vi "Gen mnu.vi"(8 "error in (no error)":errorcluster, 11 "Progress":refnum<vi>) -> (0 "error out":errorcluster, 3 "Progress (out)":refnum<vi>)   [LabVIEW 2020, in "WebServiceImporter.lvlib" / "VI Generator.lvlib"]
uses:
  <vilib>/Platform/WebService/VI Generator/VI Generator.lvlib
  <vilib>/Palette API/Palette Menu/Public Type Define/Palette type.ctl
  <vilib>/Palette API/Palette Menu/Public Type Define/Item.ctl
  <vilib>/Platform/WebService/Global/Const Strings.vi
  <resource>/importtools/Common/Icon/NISAST VI.Icon.lvclass
  <vilib>/Palette API/Palette Menu/Palette Menu.lvlib
  <vilib>/Platform/WebService/WebServiceImporter.lvlib
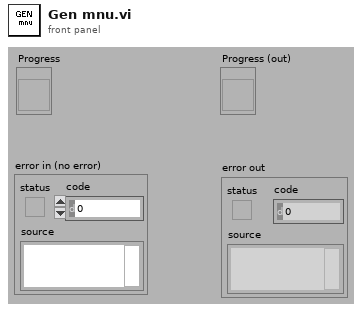
[diagram p1: front panel]
types:
  T1 = typedef "Palette Menu.lvlib/Item.ctl" = cluster{"item path":path, "library path":path, "use default lvlib palette":bool, "short name":string, "place VI contents":bool, "hide synchronized item":bool, "reserve spot for synch item":bool, "configure when placing VI contents":bool}
  T2 = typedef "Palette Menu.lvlib/Palette type.ctl" = i32
  T3 = typedef "Palette Menu.lvlib/Palette Data.ctl" = cluster{"display name":string, "view format":T4, "palette width":i16, "items":T5, "256 color icon":picture, "B&W color icon":picture, "help information":T6, "palette description":string, "synchronize information":T7}
  T4 = typedef "Palette Menu.lvlib/View Format.ctl" = u16
  T5 = typedef "Palette Menu.lvlib/Items.ctl" = T1[]
  T6 = typedef "Palette Menu.lvlib/Help Info.ctl" = cluster{"help tag":string, "help file path ":path}
  T7 = typedef "Palette Menu.lvlib/Synchronize Info.ctl" = cluster{"synchronize with directory":bool, "synchronize directory path":path}
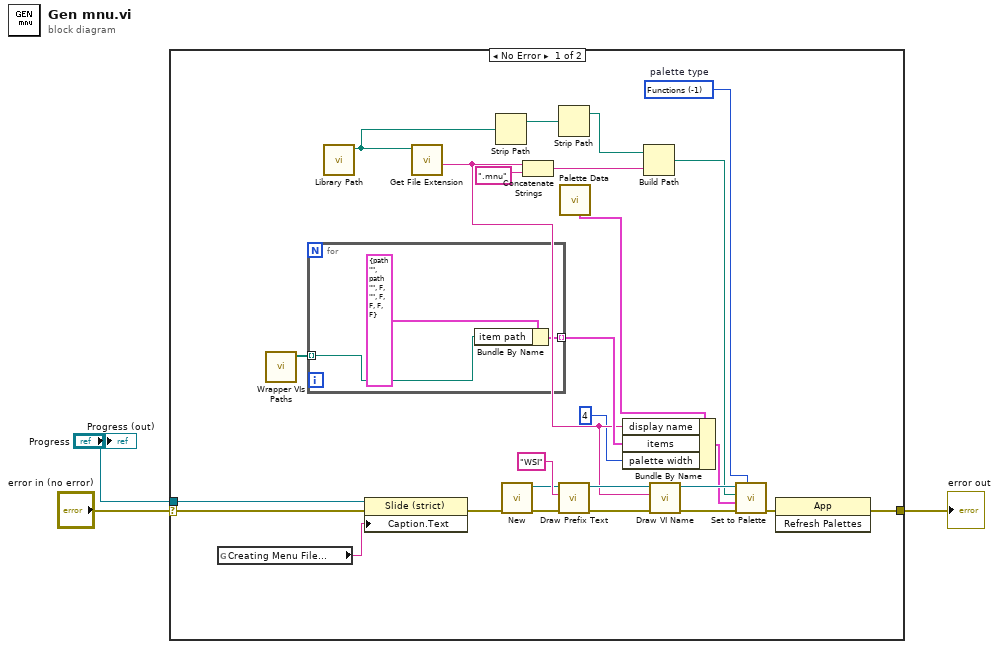
[diagram p0: block diagram]
diagram:
  n1 = case shown="No Error" "error in (no error)" {
    selector: "error in (no error)" -> [w4 w33]
    tunnel: [w14 w33] -> w3
    tunnel: "Progress" -> [w6 _]
    frame No Error {
      w16 = T2 -1 items=["Functions"=-1, "Controls"=-2]  # palette type
      n2 = global read "Const Strings.vi" "Creating Menu File..."() -> (w7:string)
      n3 = call <vilib>:"Wrapper VIs Paths.vi"() -> ("Array"=w9:path[])  [unwired: 3 in, 8 out]
      n4 = for {
        tunnel: [w32] -> w29 mode=indexing
        tunnel: w9 -> [w30] mode=indexing
        n5 = Bundle By Name(cluster=T1 {"item path"=path "", "library path"=path "", "use default lvlib palette"=FALSE, "short name"="", "place VI contents"=FALSE, "hide synchronized item"=FALSE, "reserve spot for synch item"=FALSE, "configure when placing VI contents"=FALSE} ("Items"), "item path"=w30) -> (w32:T1)
      }
      n6 = call <vilib>:"Library Path.vi"() -> ("Path (out)"=w13:path)  [unwired: 3 in, 8 out]
      n7 = property class="Slide (strict)"(reference=w6, error in=w4, "Caption.Text"=w7) -> (error out=w5:errorcluster)  [unwired: 1 out]
      n8 = call <vilib>:"Get File Extension.vi"("file"=w13) -> ("filename without extension"=w12:string)  [unwired: 1 in, 9 out]
      n9 = Strip Path(path=w13) -> (stripped path=w11:path)  [unwired: 1 out]
      n10 = call <resource>:"New.vi"("error in (no error)"=w5) -> ("error out"=w25:errorcluster, "NISAST VI.Icon out"=w21:refnum<class "NISAST VI.Icon.lvclass">)  [unwired: 1 in, 8 out]
      n11 = Concatenate Strings(w12, ".mnu" ("string")) -> (w27:string)
      n12 = Strip Path(path=w11) -> (stripped path=w10:path)  [unwired: 1 out]
      n13 = call-dynamic "Draw Prefix Text.vi"("error in (no error)"=w25, "text"="WSI", "NISAST VI.Icon in"=w21) -> ("error out"=w24:errorcluster, "NISAST VI.Icon out"=w20:refnum<class "NISAST VI.Icon.lvclass">)  [unwired: 2 in, 5 out]
      n14 = call <vilib>:"Palette Data.vi"() -> ("Palette  Data"=w28:T3)  [unwired: 11 out]
      n15 = Bundle By Name(cluster=w28, "display name"=w12, "items"=w29, "palette width"=i16 4) -> (w17:T3)
      n16 = Build Path(base path=w10, name or relative path=w27) -> (appended path=w18:path)
      n17 = call-dynamic "Draw VI Name.vi"("error in (no error)"=w24, "vi name"=w12, "NISAST VI.Icon in"=w20) -> ("error out"=w23:errorcluster, "NISAST VI.Icon out"=w19:refnum<class "NISAST VI.Icon.lvclass">)  [unwired: 3 in, 4 out]
      n18 = call-dynamic "Set to Palette.vi"("palette type"=w16, "error in (no error)"=w23, "palette data"=w17, "Palette File In"=w18, "NISAST VI.Icon in"=w19) -> ("error out"=w15:errorcluster)  [unwired: 6 out]
      n19 = invoke class="App" method="Refresh Palettes"(error in=w15) -> (error out=w14:errorcluster)  [unwired: 2 in, 2 out]
    }
    frame Error {
    }
  }
  "error out" <- w3
  "Progress (out)" <- "Progress"
